vi "Acquire Waveform.vi"(8 "error in":errorcluster, 11 "5105 in":refnum<class "5105.lvclass">) -> (0 "error out":errorcluster, 2 "wfm":waveform(dbl)[](array[waveform]), 3 "5105 out":refnum<class "5105.lvclass">)   [LabVIEW 2019, in "5105.lvlib" / "5105.lvclass"]
uses:
  5105.lvclass
  C:/Users/Public/Documents/Development/builds/Instruments/Oscilloscope.lvlibp/Oscilloscope.lvclass
  C:/Users/Public/Documents/Development/builds/Instruments/Instruments.lvlibp/Library/Instruments.lvclass
  builds/Instruments/Oscilloscope.lvlibp/Accessors/Write wfm.vi
  builds/Instruments/Instruments.lvlibp/Accessors/Write Measured with Logging.vi
  builds/Instruments/Instruments.lvlibp/Accessors/Read Measured with Logging.vi
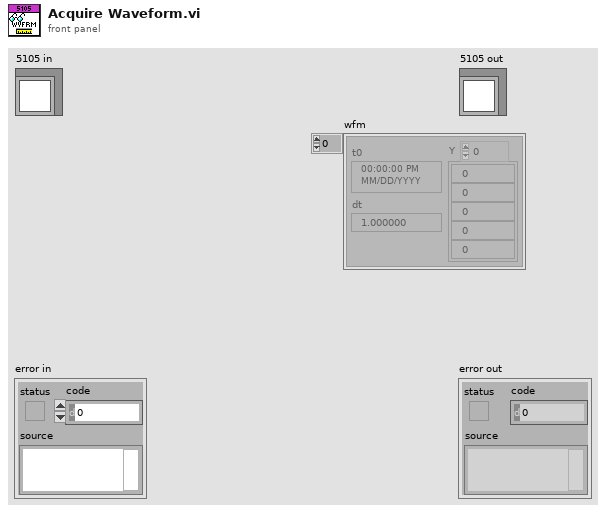
[diagram p1: front panel]
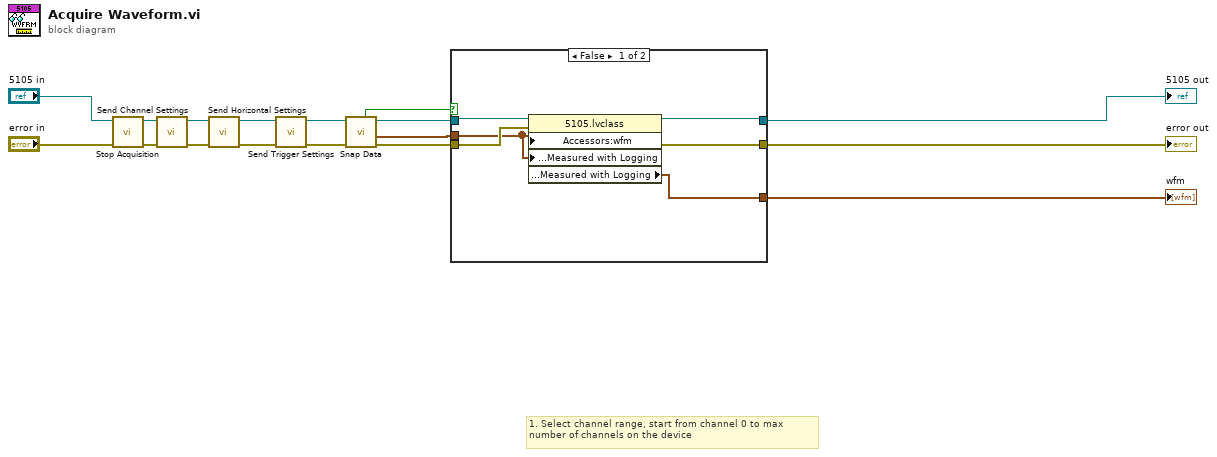
[diagram p0: block diagram]
diagram:
  # "1. Select channel range, start from channel 0 to max number of channels on the device"
  n1 = call "Stop Acquisition.vi"("error in"="error in", "5105 in"="5105 in") -> ("error out"=w2:errorcluster, "5105 out"=w3:refnum<class "5105.lvclass">)  [unwired: 8 in]
  n2 = call-dynamic "Send Channel Settings.vi"("error in"=w2, "5105 in"=w3) -> ("error out"=w17:errorcluster, "5105 out"=w16:refnum<class "5105.lvclass">)  [unwired: 8 in]
  n3 = call-dynamic "Send Horizontal Settings.vi"("error in"=w17, "5105 in"=w16) -> ("error out"=w15:errorcluster, "5105 out"=w14:refnum<class "5105.lvclass">)  [unwired: 8 in]
  n4 = call-dynamic "Send Trigger Settings.vi"("error in (no error)"=w15, "5105 in"=w14) -> ("error out"=w13:errorcluster, "5105 out"=w12:refnum<class "5105.lvclass">)  [unwired: 8 in]
  n5 = call "Snap Data.vi"("error in"=w13, "5105 in"=w12) -> ("error out"=w9:errorcluster, "wfm"=w6:waveform(dbl)[], "5105 out"=w10:refnum<class "5105.lvclass">, "Timeout"=w11:bool)  [unwired: 5 in, 1 out]
  n6 = case shown="False" w11 {
    tunnel: w10 -> [w23 w25]
    tunnel: w9 -> [w22 w24]
    tunnel: [w20 w25] -> w8
    tunnel: [w21 w24] -> w7
    tunnel: w6 -> [w19 _]
    tunnel: [w18 _] -> w5
    frame False {
      n7 = property class="5105.lvclass"(reference=w23, error in=w22, "Accessors:wfm"=w19, "Accessors:Logging:Measured with Logging"=w19) -> (reference out=w20:refnum<class "5105.lvclass">, error out=w21:errorcluster, "Accessors:Logging:Measured with Logging"=w18:waveform(dbl)[])
    }
    frame True {
    }
  }
  "error out" <- w7
  "5105 out" <- w8
  "wfm" <- w5
